vi "Init.vi"(8 "error in (no error)":errorcluster, 11 "Doña Rata Actor in":refnum<class "Doña Rata Actor.lvclass">) -> (0 "error out":errorcluster, 3 "Doña Rata Actor out":refnum<class "Doña Rata Actor.lvclass">)   [LabVIEW 2020, in "Doña Rata Actor.lvlib" / "Doña Rata Actor.lvclass"]
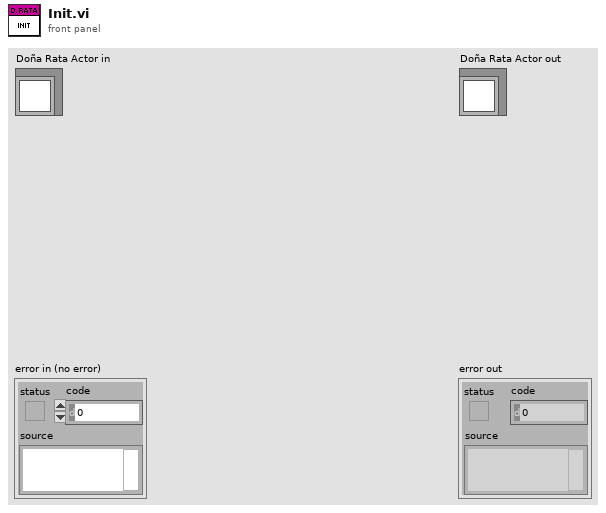
[diagram p1: front panel]
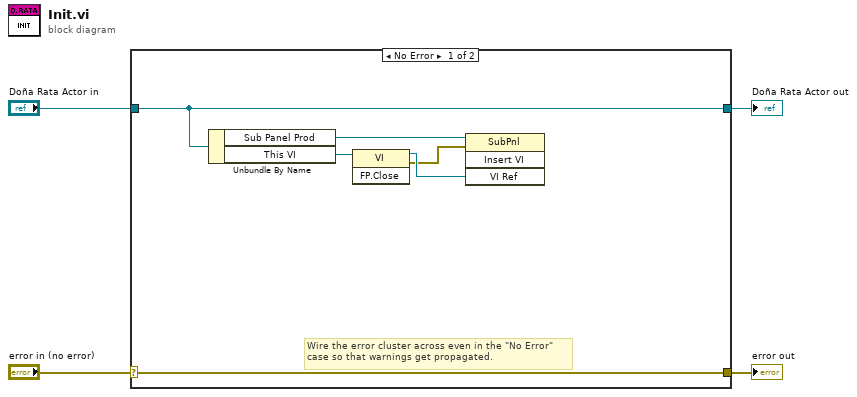
[diagram p0: block diagram]
diagram:
  n1 = case shown="No Error" "error in (no error)" {
    selector: "error in (no error)" -> [w10 w12]
    tunnel: [w10 w12] -> w3
    tunnel: [w5 w11] -> w1
    tunnel: "Doña Rata Actor in" -> [w5 w11]
    frame No Error {
      # "Wire the error cluster across even in the \"No Error\"\ncase so that warnings get propagated."
      n2 = Unbundle By Name(w5) -> ("Sub Panel Prod"=w9:refnum<vi>, "This VI"=w8:refnum<vi>)
      n3 = invoke class="VI" method="FP.Close"(reference=w8) -> (reference out=w7:refnum<vi>, error out=w6:errorcluster)  [unwired: 2 in, 1 out]
      n4 = invoke class="SubPnl" method="Insert VI"(reference=w9, error in=w6, "VI Ref"=w7) -> ()  [unwired: 1 in, 4 out]
    }
    frame Error {
    }
  }
  "error out" <- w3
  "Doña Rata Actor out" <- w1
